vi "Rec getDataToModify.vi"(4 "error in (no error)":errorcluster, 5 "ms timeout (-1)":i32=-1, 7 "recordset reference":T3) -> (0 "error out":errorcluster, 1 "timed out":bool, 2 "data":T1, 3 "recordset reference out":T3)   [LabVIEW 2013, in "NI_Database_API_64.lvlib"]
doc: "This VI returns the data associated with the <B>Recordset</B> object reference and places a lock on the object.\n\nIf the object is currently locked for modification by another method, <B>timeout</B> specifies how long the VI should wait to receive access to the object. The default value waits until the object becomes available.\n\nIf the object does not become available for modification during <B>timeout</B> milliseconds, <B>timed out</B> will return TRUE.\n\nIf, and only if, you successfully locked the object's data for modification (i.e. <B>timed out</B> returned FALSE), you must use the <B>Recordset Set Modified Data</B> VI to set the object's data and release the lock.\n\n[GOOP 1.0/1.0]"
uses:
  NI_Database_API_64.lvlib
  Rec DataMembers.ctl
  Connection.llb/Conn ObjectReference.ctl
  Rec ObjectReference.ctl
  <vilib>/Utility/_goopsup.llb/GOOP Object Repository Method.ctl
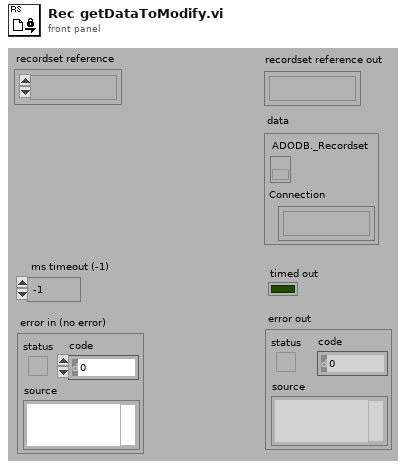
[diagram p1: front panel]
types:
  T1 = typedef "NI_Database_API_64.lvlib/Rec DataMembers.ctl" = cluster{"ADODB._Recordset":refnum<k7>, "Connection":T2}
  T2 = typedef "NI_Database_API_64.lvlib/Conn ObjectReference.ctl" = refnum<k1>
  T3 = typedef "NI_Database_API_64.lvlib/Rec ObjectReference.ctl" = refnum<k1>
  T4 = typedef "GOOP Object Repository Method.ctl" = enum16{"Create", "GetCopy", "GetModify", "Set", "Destroy", "Create Static", "Get All Refs", "Reset", "Get Statistics"}
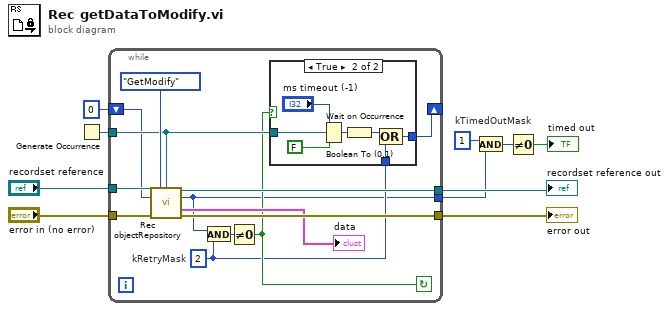
[diagram p0: block diagram]
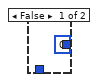
[diagram p2: hidden frame]
diagram:
  w2 = 1  # kTimedOutMask
  n1 = Generate Occurrence() -> (w4:refnum<k4>)
  n2 = while {
    tunnel: [w11] -> w1
    tunnel: w4 -> [w17]
    shift-left: 0 -> [w15]
    shift-right: [w12] -> _
    tunnel: [w22] -> w9
    tunnel: [w23] -> w7
    tunnel: "recordset reference" -> [w21]
    tunnel: "error in (no error)" -> [w20]
    stop <- w14 continue-if-true
    w13 = 2  # kRetryMask
    n3 = call "Rec objectRepository.vi"("recordset reference"=w21, "method"=GOOP_Object_Repository_Method."GetModify", "occurrence"=w17, "flags in"=w15, "error in (no error)"=w20) -> ("recordset reference out"=w23:T3, "flags out"=w11:i32, "classDataOut"=→"data":T1, "error out"=w22:errorcluster)  [unwired: 4 in, 3 out]
    n4 = And(x=w11, y=w13) -> (x .and. y?=w16:i32)
    n5 = Not Equal To 0?(x=w16) -> (x != 0?=w14:bool)
    n6 = case shown="True" w14 {
      tunnel: w17 -> [_ w29]
      tunnel: w13 -> [_ w26]
      tunnel: [0 w25] -> w12
      frame False {
      }
      frame True {
        n7 = Wait on Occurrence(1:FALSE ("ignore previous (T)"), 2:w29, 3:"ms timeout (-1)") -> (0:w27:bool)
        n8 = Boolean To (0,1)(Boolean=w27) -> (0, 1=w28:i16)
        n9 = Compound Arithmetic op=OR(w28, w26) -> (w25:i32)
      }
    }
  }
  "error out" <- w9
  "recordset reference out" <- w7
  n10 = And(x=w2, y=w1) -> (x .and. y?=w3:i32)
  n11 = Not Equal To 0?(x=w3) -> (x != 0?=→"timed out":bool)
